vi "Set Remote Heartbeat Producing Time.vi"(8 "error in":errorcluster, 11 "Network Mangement in":refnum<class "Network Mangement.lvclass">) -> (0 "error out":errorcluster, 3 "Network Mangement out":refnum<class "Network Mangement.lvclass">)   [LabVIEW 2024, in "CANopen Master.lvlib" / "Network Mangement.lvclass"]
uses:
  Network Mangement.lvclass
  Network Mangement.lvclass/Network Mangement.ctl
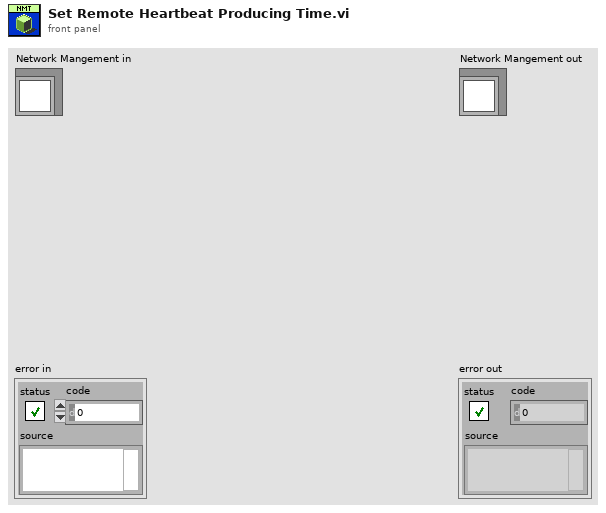
[diagram p1: front panel]
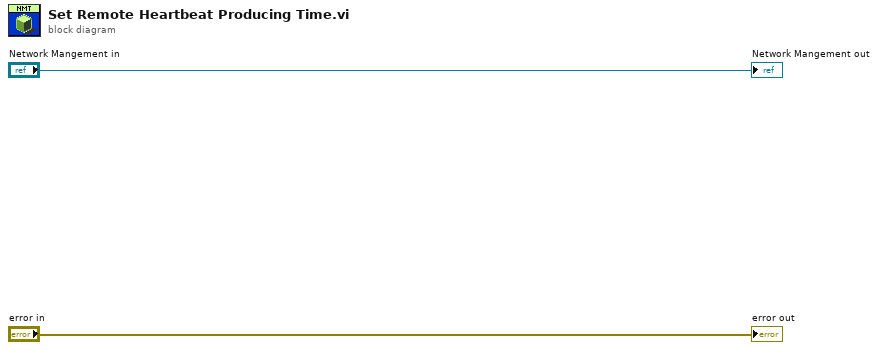
[diagram p0: block diagram]
diagram:
  "error out" <- "error in"
  "Network Mangement out" <- "Network Mangement in"
